vi "Initialise.vi"(8 "error in (no error)":errorcluster, 11 "Library Paths":T1={"SSL Library Path"=path "C:/Program Files (x86)/National Instruments/Shared/nissl/NIssleay32.dll", "Crypto Library Path"=path "C:/Program Files (x86)/National Instruments/Shared/nissl/NIlibeay32.dll"}) -> (0 "error out":errorcluster, 3 "SSL-Lib out":refnum<class "SSL-Lib.lvclass">)   [LabVIEW 2013, in "OpenSSL Socket.lvlib" / "SSL-Lib.lvclass"]
uses:
  SSL-Lib.lvclass
  Library Paths.ctl
  SSL-Lib.lvclass/SSL-Lib.ctl
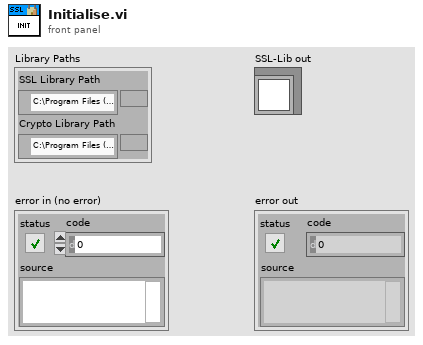
[diagram p1: front panel]
types:
  T1 = typedef "OpenSSL Socket.lvlib/SSL-Lib.lvclass/Library Paths.ctl" = cluster{"SSL Library Path":path, "Crypto Library Path":path}
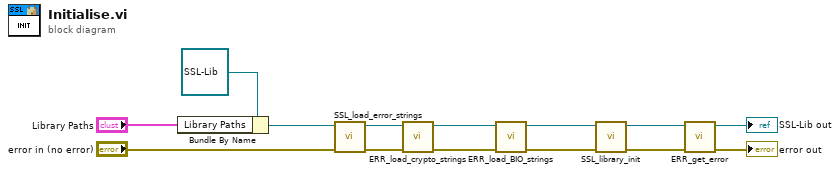
[diagram p0: block diagram]
diagram:
  n1 = Bundle By Name(cluster=refnum<class "SSL-Lib.lvclass"> refnum ("SSL-Lib in"), "Library Paths"="Library Paths") -> (w1:refnum<class "SSL-Lib.lvclass">)
  n2 = call "SSL_load_error_strings.vi"("error in (no error)"="error in (no error)", "SSL-Lib in"=w1) -> ("error out"=w9:errorcluster, "SSL-Lib out"=w12:refnum<class "SSL-Lib.lvclass">)  [unwired: 8 in]
  n3 = call "ERR_load_crypto_strings.vi"("error in (no error)"=w9, "SSL-Lib in"=w12) -> ("error out"=w10:errorcluster, "SSL-Lib out"=w13:refnum<class "SSL-Lib.lvclass">)  [unwired: 8 in]
  n4 = call "ERR_load_BIO_strings.vi"("error in (no error)"=w10, "SSL-Lib in"=w13) -> ("error out"=w11:errorcluster, "SSL-Lib out"=w14:refnum<class "SSL-Lib.lvclass">)  [unwired: 8 in]
  n5 = call "SSL_library_init.vi"("error in (no error)"=w11, "SSL-Lib in"=w14) -> ("error out"=w6:errorcluster, "SSL-Lib out"=w5:refnum<class "SSL-Lib.lvclass">)  [unwired: 8 in]
  n6 = call "ERR_get_error.vi"("error in (no error)"=w6, "SSL-Lib in"=w5) -> ("error out"=→"error out":errorcluster, "SSL-Lib out"=→"SSL-Lib out":refnum<class "SSL-Lib.lvclass">)  [unwired: 8 in]
